vi "Assert Selection.vi"(9 "Actual":T1, 10 "Expected":T1, 11 "Added Section Finder Test In":refnum<class "Diff Tool Test.lvclass">) -> (0 "error out":errorcluster, 3 "Added Section Finder Test Out":refnum<class "Diff Tool Test.lvclass">)   [LabVIEW 2020, in "Diff Tool Test.lvclass"]
uses:
  Diff Tool Test.lvclass
  usr/local/natinst/LabVIEW-2026-64/vi.lib/Astemes/LUnit/Test Case.lvclass
  <vilib>/Astemes/LUnit/Test Case.lvclass/Test Case.ctl
  <vilib>/Astemes/LUnit/Test Case.lvclass
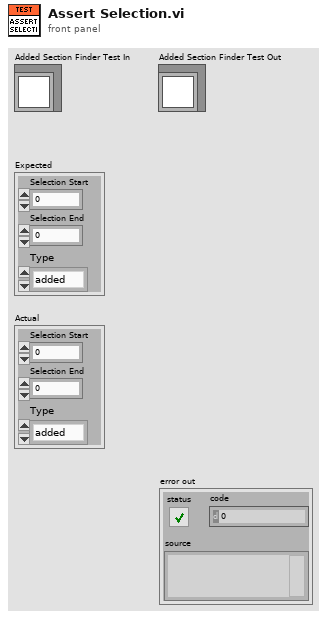
[diagram p1: front panel]
types:
  T1 = cluster{"Selection Start":u32, "Selection End":u32, "Type":enum16{"added", "missing"}}
  T2 = cluster{"Selection Start":bool, "Selection End":bool, "Type":bool}
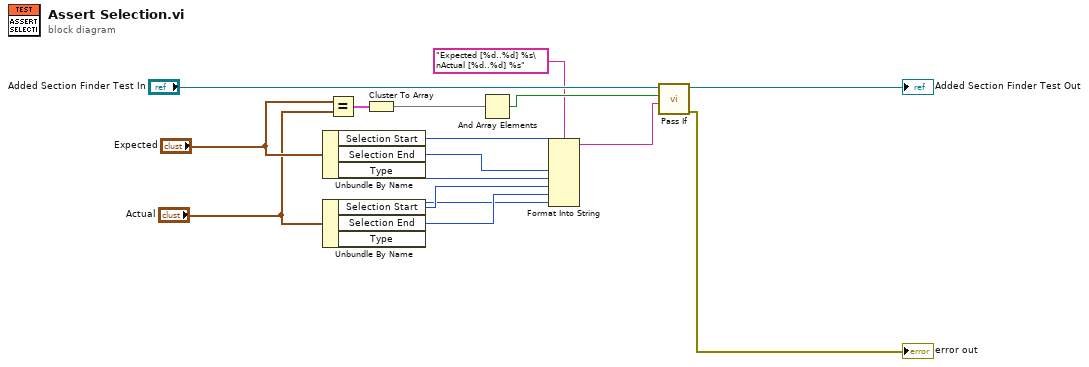
[diagram p0: block diagram]
diagram:
  n1 = Unbundle By Name("Expected") -> ("Selection Start"=w7:u32, "Selection End"=w6:u32, "Type"=w2:enum16{"added", "missing"})
  n2 = Unbundle By Name("Actual") -> ("Selection Start"=w5:u32, "Selection End"=w4:u32, "Type"=w1:enum16{"added", "missing"})
  n3 = Equal?(x="Expected", y="Actual") -> (x = y?=w11:T2)
  n4 = Cluster To Array(cluster=w11) -> (array=w10:bool[])
  n5 = And Array Elements(Boolean array=w10) -> (logical AND=w9:bool)
  n6 = Format Into String(format string="Expected [%d..%d] %s\nActual [%d..%d] %s", w7, w6, w2, w5, w4, w1) -> (resulting string=w3:string)  [unwired: 2 in, 1 out]
  n7 = call <vilib>:"Pass If.vi"("Message"=w3, "Pass?"=w9, "LUnit Test Case In"="Added Section Finder Test In") -> ("error out"=→"error out":errorcluster, "LUnit Test Case Out"=→"Added Section Finder Test Out":refnum<class "Diff Tool Test.lvclass">)  [unwired: 7 in]
